vi "Page_Info_Initialize.vi"(8 "error in (no error)":errorcluster, 9 "ctlReferences":T1, 11 "AB_Targetfile in":refnum<class "AB_Targetfile.lvclass">) -> (0 "error out":errorcluster, 3 "AB_Targetfile out":refnum<class "AB_Targetfile.lvclass">)   [LabVIEW 2020, in "AB_Targetfile.lvclass"]
uses:
  <vilib>/AppBuilder/AB_Classes/TargetFile/AB_Targetfile.lvclass
  <resource>/Framework/Providers/Builds/AppBuilder/AB_UI_Page_Info_References.ctl
  <resource>/Framework/Providers/Common/provcom_StringGlobals.vi
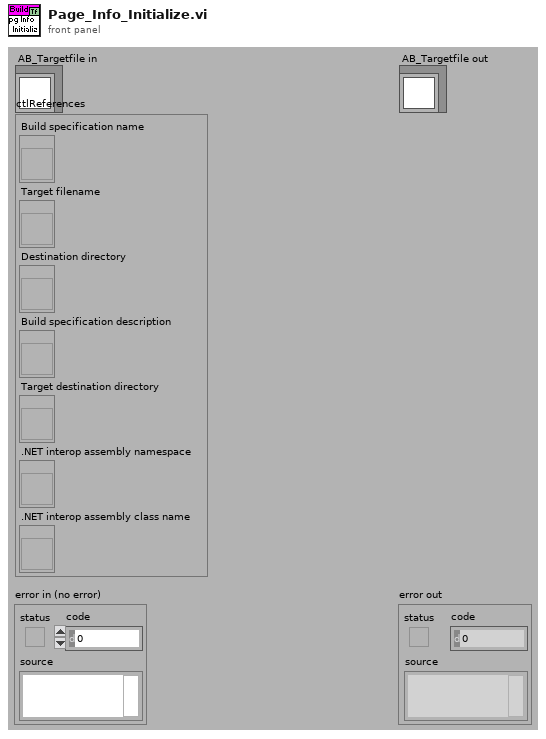
[diagram p1: front panel]
types:
  T1 = typedef "AB_UI_Page_Info_References.ctl" = cluster{"Build specification name":refnum<vi>, "Target filename":refnum<vi>, "Destination directory":refnum<vi>, "Build specification description":refnum<vi>, "Target destination directory":refnum<vi>, ".NET interop assembly namespace":refnum<vi>, ".NET interop assembly class name":refnum<vi>}
  T2 = typedef "LVRectTypeDef.ctl" = cluster{"Left":i16, "Top":i16, "Right":i16, "Bottom":i16}
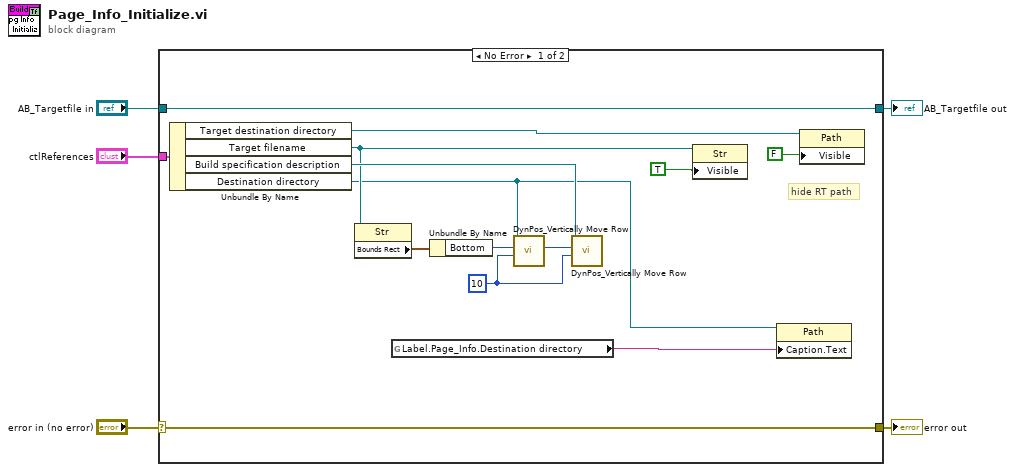
[diagram p0: block diagram]
diagram:
  n1 = case shown="No Error" "error in (no error)" {
    selector: "error in (no error)" -> [w17 w21]
    tunnel: [w17 w21] -> w2
    tunnel: [w18 w20] -> w4
    tunnel: "AB_Targetfile in" -> [w18 w20]
    tunnel: "ctlReferences" -> [w19 _]
    frame No Error {
      w13 = 10 ("Pixel separation (6)")
      # "hide RT path"
      n2 = Unbundle By Name(w19) -> ("Target destination directory"=w8:refnum<vi>, "Target filename"=w10:refnum<vi>, "Build specification description"=w12:refnum<vi>, "Destination directory"=w6:refnum<vi>)
      n3 = property class="Str"(reference=w10) -> ("Bounds Rect"=w16:T2)  [unwired: 1 in, 2 out]
      n4 = global read "provcom_StringGlobals.vi" "Label.Page_Info.Destination directory"() -> (w7:string)
      n5 = Unbundle By Name(w16) -> ("Bottom"=w15:i16)
      n6 = call <vilib>:"DynPos_Vertically Move Row.vi"("Pixel separation (6)"=w13, "Bottom of last control"=w15, "Control"=w6) -> ("Bottom pixel"=w14:i32)  [unwired: 7 in, 1 out]
      n7 = call <vilib>:"DynPos_Vertically Move Row.vi"("Pixel separation (6)"=w13, "Bottom of last control"=w14, "Control"=w12) -> ()  [unwired: 7 in, 2 out]
      n8 = property class="Str"(reference=w10, "Visible"=TRUE) -> ()  [unwired: 1 in, 2 out]
      n9 = property class="Path"(reference=w6, "Caption.Text"=w7) -> ()  [unwired: 1 in, 2 out]
      n10 = property class="Path"(reference=w8, "Visible"=FALSE) -> ()  [unwired: 1 in, 2 out]
    }
    frame Error {
    }
  }
  "error out" <- w2
  "AB_Targetfile out" <- w4
